vi "Enable Output.vi"(8 "error in (no error)":errorcluster, 10 "Output Enable (F)":bool, 11 "SigGen-8665B in":refnum<class "SigGen-8665B.lvclass">) -> (0 "error out":errorcluster, 3 "SigGen-8665B out":refnum<class "SigGen-8665B.lvclass">)   [LabVIEW 2020, in "SigGen-8665B.lvclass"]
uses:
  SigGen-8665B.lvclass
  C:/Sandbox/RF Bench/Source Code/WiSpry Test Framework/Instruments/Instrument.lvclass
  Instrument.lvclass/Instrument.ctl
  Instrument.lvclass
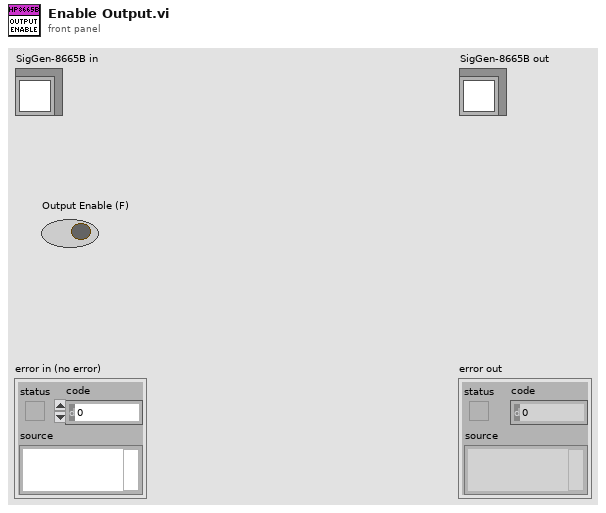
[diagram p1: front panel]
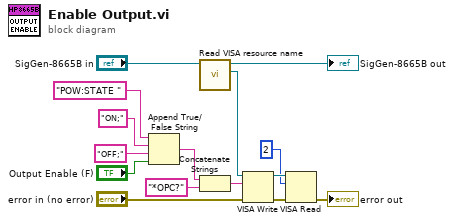
[diagram p0: block diagram]
diagram:
  n1 = Append True/False String(1:"Output Enable (F)", 2:"OFF;" ("false string"), 3:"ON;" ("true string"), 4:"POW:STATE " ("true string")) -> (0:w10:string)
  n2 = call "Read VISA resource name.vi"("Instrument in"="SigGen-8665B in") -> ("VISA resource name"=w8:refnum<visa-resource-name>, "Instrument out"=→"SigGen-8665B out":refnum<class "SigGen-8665B.lvclass">)  [unwired: 9 in]
  n3 = Concatenate Strings(w10, "*OPC?" ("string")) -> (w6:string)
  n4 = VISA Write(VISA resource name=w8, write buffer=w6, error in (no error)="error in (no error)") -> (VISA resource name out=w4:refnum<visa-resource-name>, error out=w5:errorcluster)  [unwired: 1 out]
  n5 = VISA Read(VISA resource name=w4, byte count=u32 2, error in (no error)=w5) -> (error out=→"error out":errorcluster)  [unwired: 3 out]
